vi "tutorial4_traficlight.vi"() -> ()   [LabVIEW 2020]
panel:
  out "Numeric":dbl
  out "Status C":bool
  out "Status B":bool
  out "Status A":bool
  out "Green  5":bool
  out "Yellow   5":bool
  out "Red  5":bool
  out "Green  4":bool
  out "Yellow   4":bool
  out "Red  4":bool
  out "Green  3":bool
  out "Yellow   3":bool
  out "Red  3":bool
  out "Green  2":bool
  out "Yellow   2":bool
  out "Red  2":bool
  # "C"
  # "D"
  # "A"
  # "B"
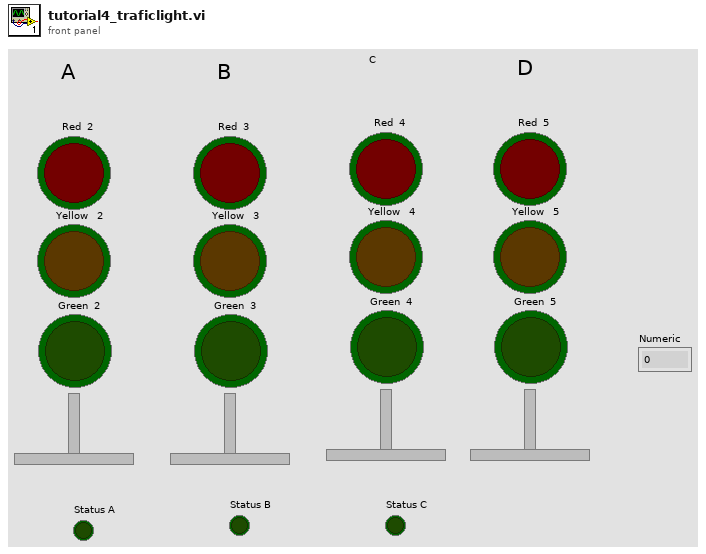
[diagram p1: front panel]
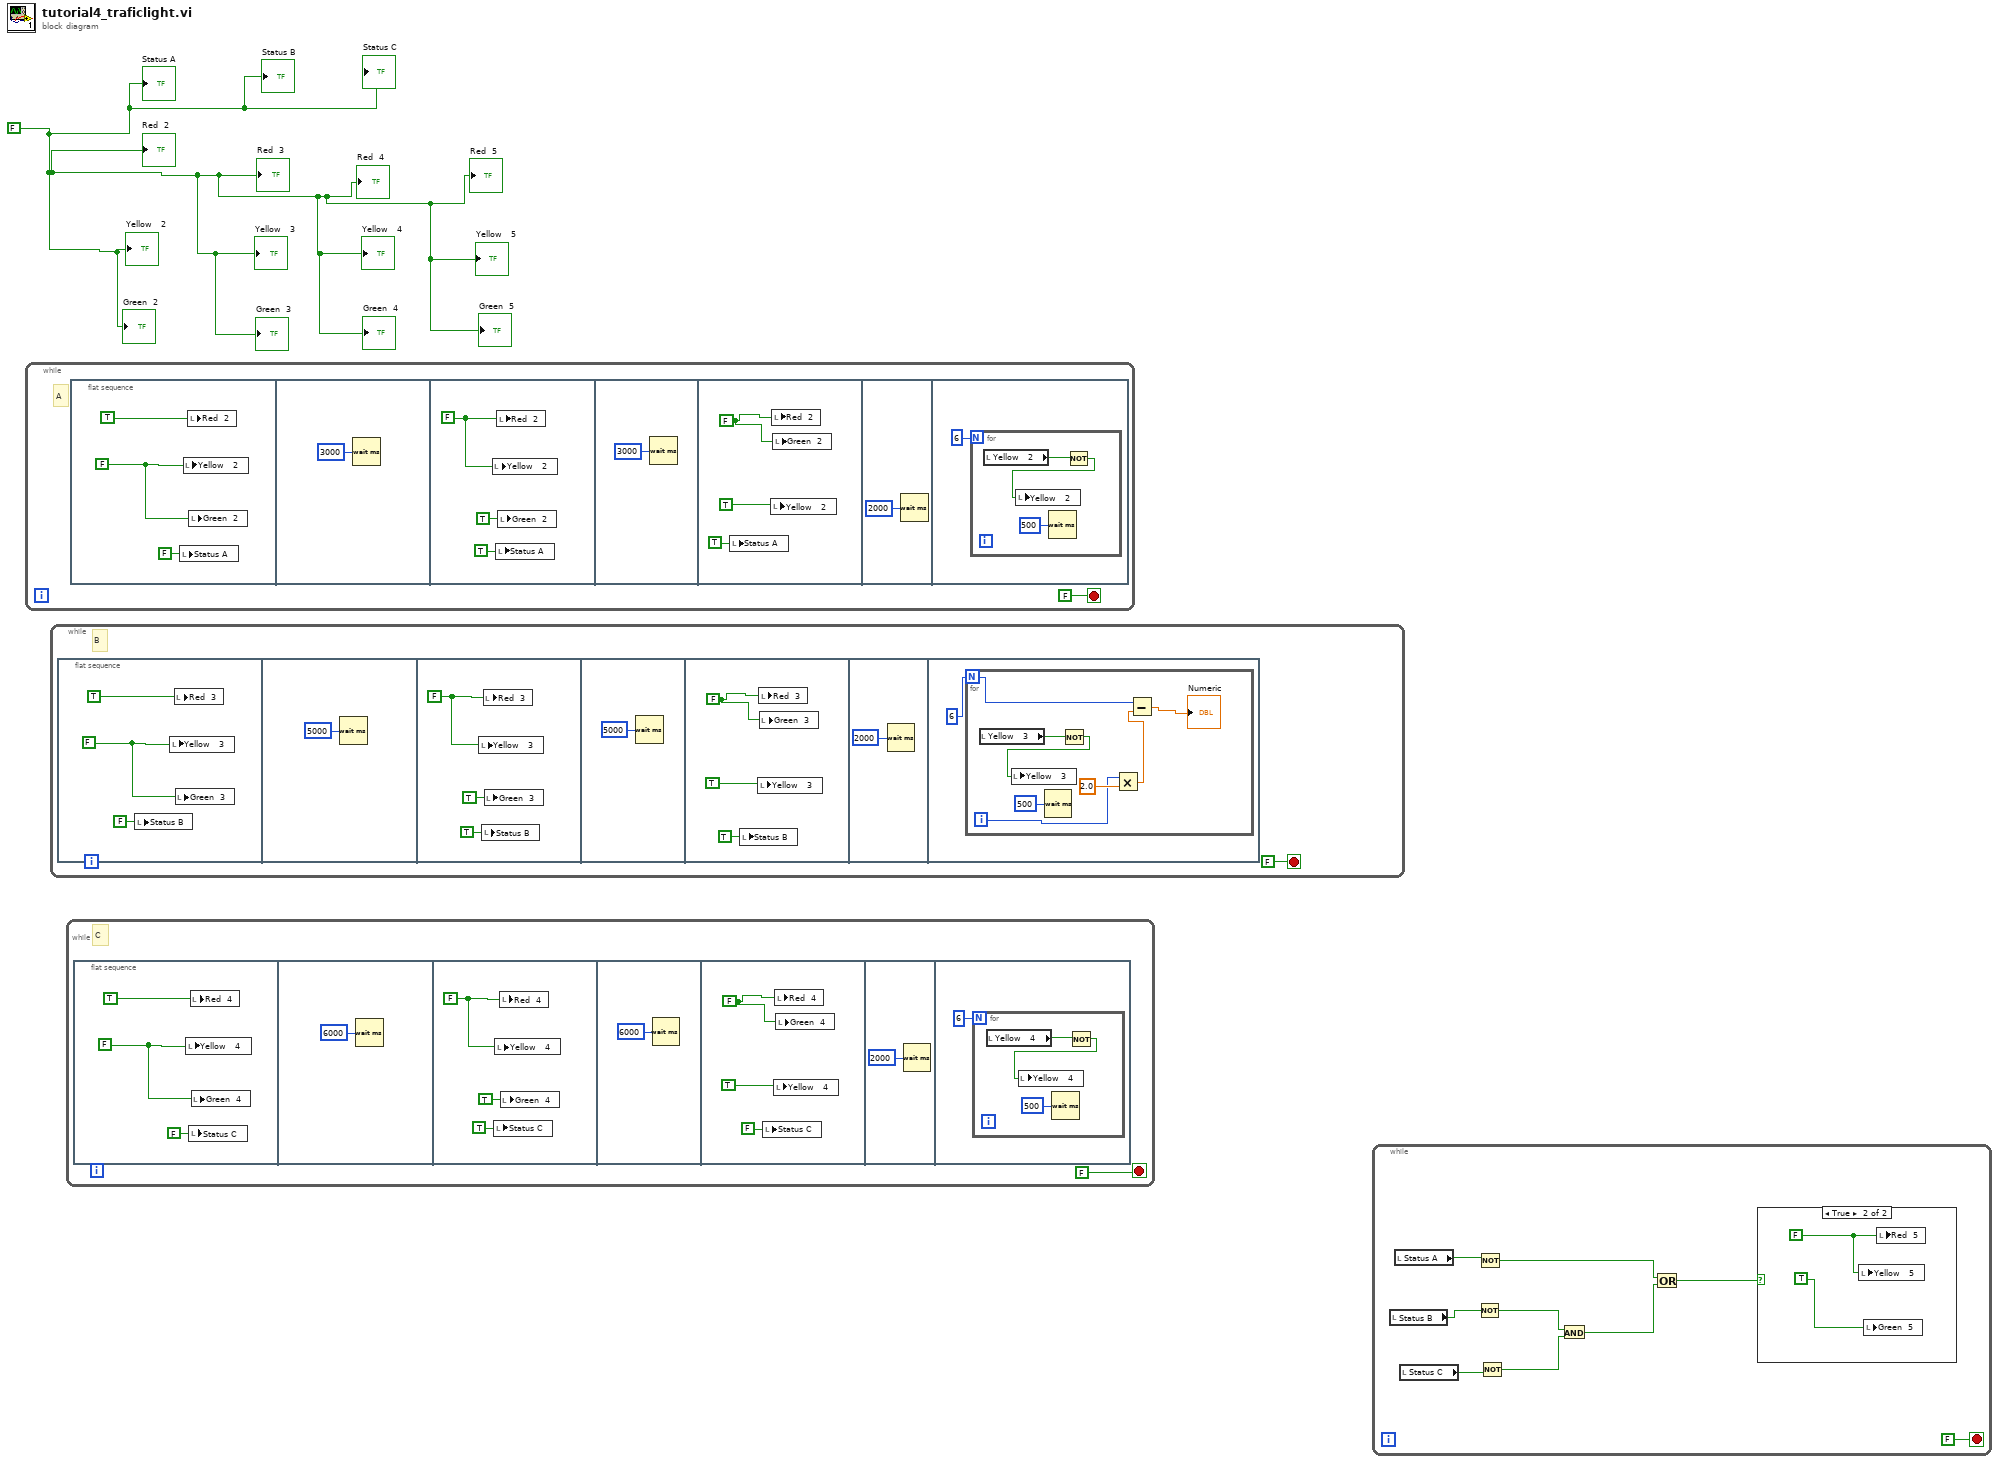
[diagram p0: block diagram]
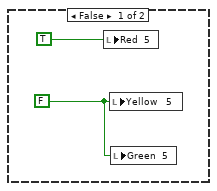
[diagram p2: hidden frame]
diagram:
  w1 = FALSE
  n1 = while {
    stop <- FALSE stop-if-true
    # "A"
    n2 = flat-sequence {
      frame #0 {
        w4 = FALSE ("Yellow   2")
        n3 = local write "Status A"(FALSE ("Status A")) -> ()
        n4 = local write "Yellow   2"(w4) -> ()
        n5 = local write "Red  2"(TRUE) -> ()
        n6 = local write "Green  2"(w4) -> ()
      }
      frame #1 {
        n7 = Wait (ms)(milliseconds to wait=u32 3000) -> ()  [unwired: 1 out]
      }
      frame #2 {
        w8 = FALSE ("Red  2")
        n8 = local write "Yellow   2"(w8) -> ()
        n9 = local write "Status A"(TRUE ("Status A")) -> ()
        n10 = local write "Red  2"(w8) -> ()
        n11 = local write "Green  2"(TRUE ("Green  2")) -> ()
      }
      frame #3 {
        n12 = Wait (ms)(milliseconds to wait=u32 3000) -> ()  [unwired: 1 out]
      }
      frame #4 {
        w13 = FALSE
        n13 = local write "Status A"(TRUE ("Status A")) -> ()
        n14 = local write "Yellow   2"(TRUE) -> ()
        n15 = local write "Red  2"(w13) -> ()
        n16 = local write "Green  2"(w13) -> ()
      }
      frame #5 {
        n17 = Wait (ms)(milliseconds to wait=u32 2000) -> ()  [unwired: 1 out]
      }
      frame #6 {
        n18 = for {
          N: 6 -> [_]
          n19 = local read "Yellow   2"() -> (w17:bool)
          n20 = Wait (ms)(milliseconds to wait=u32 500) -> ()  [unwired: 1 out]
          n21 = Not(x=w17) -> (.not. x?=w16:bool)
          n22 = local write "Yellow   2"(w16) -> ()
        }
      }
    }
  }
  n23 = while {
    stop <- FALSE stop-if-true
    # "B"
    n24 = flat-sequence {
      frame #0 {
        w21 = FALSE ("Yellow   2")
        n25 = local write "Status B"(FALSE ("Status B")) -> ()
        n26 = local write "Yellow   3"(w21) -> ()
        n27 = local write "Red  3"(TRUE) -> ()
        n28 = local write "Green  3"(w21) -> ()
      }
      frame #1 {
        n29 = Wait (ms)(milliseconds to wait=u32 5000) -> ()  [unwired: 1 out]
      }
      frame #2 {
        w25 = FALSE ("Red  2")
        n30 = local write "Yellow   3"(w25) -> ()
        n31 = local write "Status B"(TRUE ("Status B")) -> ()
        n32 = local write "Red  3"(w25) -> ()
        n33 = local write "Green  3"(TRUE ("Green  2")) -> ()
      }
      frame #3 {
        n34 = Wait (ms)(milliseconds to wait=u32 5000) -> ()  [unwired: 1 out]
      }
      frame #4 {
        w30 = FALSE
        n35 = local write "Status B"(TRUE ("Status B")) -> ()
        n36 = local write "Yellow   3"(TRUE) -> ()
        n37 = local write "Red  3"(w30) -> ()
        n38 = local write "Green  3"(w30) -> ()
      }
      frame #5 {
        n39 = Wait (ms)(milliseconds to wait=u32 2000) -> ()  [unwired: 1 out]
      }
      frame #6 {
        n40 = for {
          N: 6 -> [w37]
          i -> [w35]
          n41 = local read "Yellow   3"() -> (w39:bool)
          n42 = Wait (ms)(milliseconds to wait=u32 500) -> ()  [unwired: 1 out]
          n43 = Not(x=w39) -> (.not. x?=w38:bool)
          n44 = local write "Yellow   3"(w38) -> ()
          n45 = Multiply(x=w35, y=2.0) -> (x*y=w34:dbl)
          n46 = Subtract(x=w37, y=w34) -> (x-y=→"Numeric":dbl)
        }
      }
    }
  }
  n47 = while {
    stop <- FALSE stop-if-true
    # "C"
    n48 = flat-sequence {
      frame #0 {
        w43 = FALSE ("Yellow   2")
        n49 = local write "Yellow   4"(w43) -> ()
        n50 = local write "Status C"(FALSE ("Status C")) -> ()
        n51 = local write "Red  4"(TRUE) -> ()
        n52 = local write "Green  4"(w43) -> ()
      }
      frame #1 {
        n53 = Wait (ms)(milliseconds to wait=u32 6000) -> ()  [unwired: 1 out]
      }
      frame #2 {
        w47 = FALSE ("Red  2")
        n54 = local write "Status C"(TRUE ("Status C")) -> ()
        n55 = local write "Yellow   4"(w47) -> ()
        n56 = local write "Red  4"(w47) -> ()
        n57 = local write "Green  4"(TRUE ("Green  2")) -> ()
      }
      frame #3 {
        n58 = Wait (ms)(milliseconds to wait=u32 6000) -> ()  [unwired: 1 out]
      }
      frame #4 {
        w52 = FALSE
        n59 = local write "Status C"(FALSE ("Status C")) -> ()
        n60 = local write "Yellow   4"(TRUE) -> ()
        n61 = local write "Red  4"(w52) -> ()
        n62 = local write "Green  4"(w52) -> ()
      }
      frame #5 {
        n63 = Wait (ms)(milliseconds to wait=u32 2000) -> ()  [unwired: 1 out]
      }
      frame #6 {
        n64 = for {
          N: 6 -> [_]
          n65 = local read "Yellow   4"() -> (w56:bool)
          n66 = Wait (ms)(milliseconds to wait=u32 500) -> ()  [unwired: 1 out]
          n67 = Not(x=w56) -> (.not. x?=w55:bool)
          n68 = local write "Yellow   4"(w55) -> ()
        }
      }
    }
  }
  n69 = while {
    stop <- FALSE stop-if-true
    n70 = local read "Status B"() -> (w60:bool)
    n71 = local read "Status A"() -> (w61:bool)
    n72 = local read "Status C"() -> (w59:bool)
    n73 = Not(x=w60) -> (.not. x?=w66:bool)
    n74 = Not(x=w61) -> (.not. x?=w64:bool)
    n75 = Not(x=w59) -> (.not. x?=w65:bool)
    n76 = And(x=w66, y=w65) -> (x .and. y?=w63:bool)
    n77 = Or(x=w64, y=w63) -> (x .or. y?=w62:bool)
    n78 = case shown="True" w62 {
      frame False {
        w67 = FALSE ("Yellow   5")
        n79 = local write "Red  5"(TRUE ("Red  5")) -> ()
        n80 = local write "Yellow   5"(w67) -> ()
        n81 = local write "Green  5"(w67) -> ()
      }
      frame True {
        w69 = FALSE ("Red  5")
        n82 = local write "Yellow   5"(w69) -> ()
        n83 = local write "Green  5"(TRUE ("Yellow   5")) -> ()
        n84 = local write "Red  5"(w69) -> ()
      }
    }
  }
  "Red  2" <- w1
  "Yellow   2" <- w1
  "Green  2" <- w1
  "Red  3" <- w1
  "Yellow   3" <- w1
  "Green  3" <- w1
  "Red  4" <- w1
  "Yellow   4" <- w1
  "Green  4" <- w1
  "Red  5" <- w1
  "Yellow   5" <- w1
  "Green  5" <- w1
  "Status A" <- w1
  "Status B" <- w1
  "Status C" <- w1
